vi "Get Error Handling Parameters.vi"(4 "Error In":errorcluster) -> (0 "Error Out":errorcluster, 1 "Stop Button":string, 2 "Continue/Ok Button":string, 3 "Action":T1(ring)=enum."Ok Only")   [LabVIEW 2014, in "Config Data.lvlib" / "Config Data.lvclass"]
uses:
  Config Data.lvclass
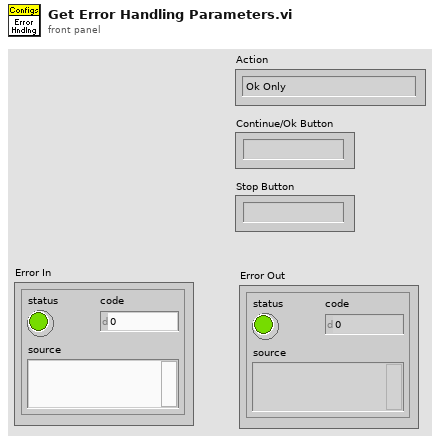
[diagram p1: front panel]
types:
  T1 = enum16{"Ok + Logging", "Continue/Stop + Logging", "Logging Only", "Ok Only", "Continue/Stop Only"}
  T2 = cluster{"Continue/Ok Button":string, "Stop Button":string}
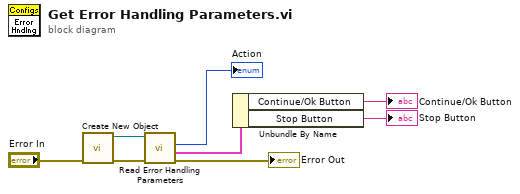
[diagram p0: block diagram]
diagram:
  n1 = call "Create New Object.vi"("Error In"="Error In") -> ("Error Out"=w6:errorcluster, "Config Data"=w7:refnum<class "Config Data.lvclass">)  [unwired: 5 in]
  n2 = call-dynamic "Read Error Handling Parameters.vi"("Error In"=w6, "Config Data in"=w7) -> ("Error Out"=→"Error Out":errorcluster, "Buttons"=w3:T2, "Action"=→"Action":T1)  [unwired: 2 in, 1 out]
  n3 = Unbundle By Name(w3) -> ("Continue/Ok Button"=→"Continue/Ok Button":string, "Stop Button"=→"Stop Button":string)
